vi "Channel Load.vi"   [LabVIEW 2020, in "G-Audio.lvlib" / "Mixer.lvclass"]
doc: "<b>This VI is polymorphic.</b>\n\nReads an audio file into memory, and associates it with a channel.\n\n<b>Path</b> can be a standard path type, or a UTF-8 encoded string.\n\nWhen <b>Wait For Load</b> is true, this VI blocks until the audio file has been loaded into a channel. If <b>Wait For Load</b> is false, this VI returns immediately and the audio file is loaded asynchronously in the background. The channel will be in a Loading state while the file is read, and then set to Loaded once the load is complete, or Empty if there was an error."
uses:
  Mixer.lvclass
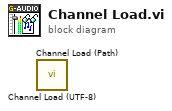
[diagram p0: block diagram]
diagram:
  n1 = call "Channel Load (UTF-8).vi"() -> ()  [unwired: 10 in, 2 out]
  n2 = call "Channel Load (Path).vi"() -> ()  [unwired: 10 in, 2 out]
